vi "SIM limit signal (array).vi"(6 "lower limits":dbl[](array[numeric]) format="%.2f", 7 "upper limits":dbl[](array[numeric]) format="%.2f", 9 "limit types":T1[](array[typedef]), 10 "limited? in":bool[](array[boolean]), 11 "inputs":dbl[](array[numeric]) format="%.2f") -> (2 "limited? out":bool[](array[boolean]), 3 "outputs":dbl[](array[numeric]) format="%.2f")   [LabVIEW 2020]
uses:
  <vilib>/Simulation/Implementation/Shared/SIM limit type.ctl
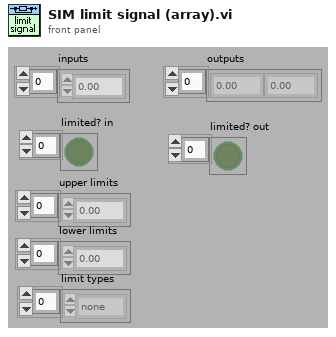
[diagram p1: front panel]
types:
  T1 = typedef "SIM limit type.ctl" = enum16{"upper", "lower", "both", "none"}
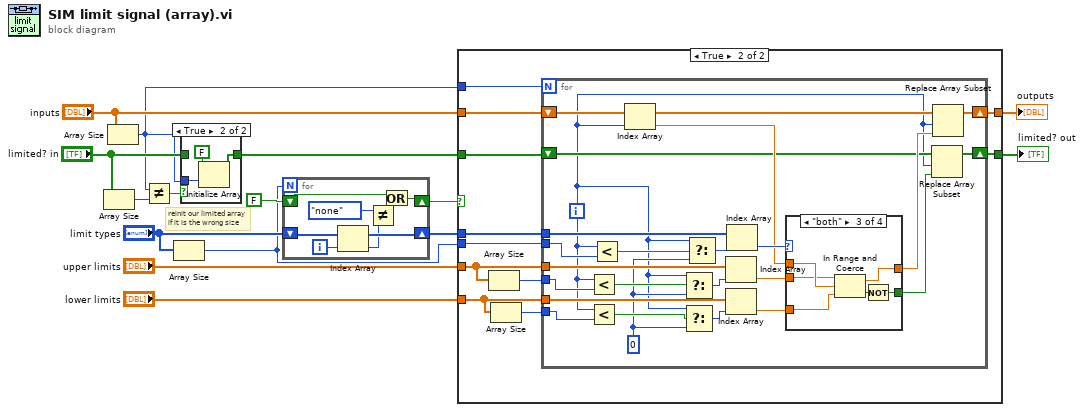
[diagram p0: block diagram]
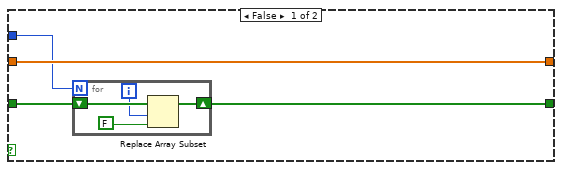
[diagram p3: hidden frame]
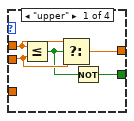
[diagram p4: hidden frame]
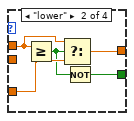
[diagram p5: hidden frame]
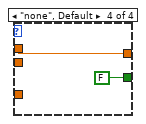
[diagram p6: hidden frame]
diagram:
  # "reinit our limited array\nif it is the wrong size"
  n1 = Array Size(array="limited? in") -> (size(s)=w7:i32)
  n2 = Array Size(array="inputs") -> (size(s)=w1:i32)
  n3 = Not Equal?(x=w1, y=w7) -> (x != y?=w6:bool)
  n4 = Array Size(array="limit types") -> (size(s)=w3:i32)
  n5 = case shown="True" w6 {
    tunnel: "limited? in" -> [w16 _]
    tunnel: w1 -> [_ w19]
    tunnel: [w16 w17] -> w2
    frame False {
    }
    frame True {
      n6 = Initialize Array(FALSE, w19) -> (w17:bool[])
    }
  }
  n7 = for {
    N: w3 -> [_]
    shift-right: [w26] -> w11
    shift-left: "limit types" -> [w26]
    shift-right: [w21] -> w10
    shift-left: FALSE -> [w23]
    i -> [w20]
    n8 = Index Array(array=w26, index=w20) -> (element=w24:T1)
    n9 = Not Equal?(x=SIM_limit_type."none" ("limit type"), y=w24) -> (x != y?=w22:bool)
    n10 = Or(x=w23, y=w22) -> (x .or. y?=w21:bool)
  }
  n11 = case shown="True" w10 {
    tunnel: "upper limits" -> [_ w45]
    tunnel: "lower limits" -> [_ w44]
    tunnel: [w30 w38] -> w13
    tunnel: "inputs" -> [w30 w39]
    tunnel: w11 -> [_ w41]
    tunnel: w2 -> [w29 w37]
    tunnel: [w27 w40] -> w9
    tunnel: w3 -> [_ w36]
    tunnel: w1 -> [w28 w35]
    frame False {
      n12 = for {
        N: w28 -> [_]
        shift-right: [w31] -> w27
        shift-left: w29 -> [w34]
        i -> [w32]
        n13 = Replace Array Subset(array=w34, new element=FALSE ("new element/subarray"), index=w32) -> (w31:bool[])
      }
    }
    frame True {
      n14 = Array Size(array=w45) -> (size(s)=w43:i32)
      n15 = Array Size(array=w44) -> (size(s)=w42:i32)
      n16 = for {
        N: w35 -> [_]
        tunnel: w45 -> [w65]
        tunnel: w44 -> [w64]
        tunnel: w41 -> [w63]
        tunnel: w36 -> [w48]
        tunnel: w43 -> [w49]
        tunnel: w42 -> [w50]
        shift-right: [w55] -> w40
        shift-left: w37 -> [w51]
        shift-right: [w53] -> w38
        shift-left: w39 -> [w54]
        i -> [w46]
        w62 = 0
        n17 = Less?(x=w46, y=w49) -> (x < y?=w68:bool)
        n18 = Less?(x=w46, y=w50) -> (x < y?=w67:bool)
        n19 = Less?(x=w46, y=w48) -> (x < y?=w61:bool)
        n20 = Index Array(array=w54, index=w46) -> (element=w58:dbl)
        n21 = Select(t=w46, s=w68, f=w62) -> (s? t:f=w69:i32)
        n22 = Select(t=w46, s=w67, f=w62) -> (s? t:f=w66:i32)
        n23 = Select(t=w46, s=w61, f=w62) -> (s? t:f=w47:i32)
        n24 = Index Array(array=w65, index=w69) -> (element=w59:dbl)
        n25 = Index Array(array=w64, index=w66) -> (element=w57:dbl)
        n26 = Index Array(array=w63, index=w47) -> (element=w60:T1)
        n27 = case shown="\"both\"" w60 {
          tunnel: [w74 w79 w85 w87] -> w52
          tunnel: w59 -> [w72 _ w83 _]
          tunnel: w58 -> [w73 w78 w84 w87]
          tunnel: w57 -> [_ w77 w82 _]
          tunnel: [w70 w75 w80 FALSE] -> w56
          frame "upper" {
            n28 = Less Or Equal?(x=w73, y=w72) -> (x <= y?=w71:bool)
            n29 = Select(t=w73, s=w71, f=w72) -> (s? t:f=w74:dbl)
            n30 = Not(x=w71) -> (.not. x?=w70:bool)
          }
          frame "lower" {
            n31 = Greater Or Equal?(x=w78, y=w77) -> (x >= y?=w76:bool)
            n32 = Select(t=w78, s=w76, f=w77) -> (s? t:f=w79:dbl)
            n33 = Not(x=w76) -> (.not. x?=w75:bool)
          }
          frame "both" {
            n34 = In Range and Coerce(upper limit=w83, x=w84, lower limit=w82) -> (coerced(x)=w85:dbl, In Range?=w81:bool)
            n35 = Not(x=w81) -> (.not. x?=w80:bool)
          }
          frame "none", Default {
            (unwired) TRUE
          }
        }
        n36 = Replace Array Subset(array=w51, new element=w56, index=w46) -> (w55:bool[])
        n37 = Replace Array Subset(array=w54, new element=w52, index=w46) -> (w53:dbl[])
      }
    }
  }
  "outputs" <- w13
  "limited? out" <- w9
